vi "Robot Global Data.vi"() -> ()   [LabVIEW 2015]
doc: "This global VI can contain as many global variables as you need. Place a control on the panel, give it a good name. To read or write to it from a VI, drag the icon to the diagram of that VI. You can also drag from the project. Click on the node to change which global you access. You shouldn't have multiple locations writing to a global or it will cause a race-condition."
uses:
  <vilib>/Rock Robotics/WPI/Camera/WPI_CameraImageSize.ctl
  <vilib>/Rock Robotics/WPI/DriverStation/WPI_DriverStationRobotMode2.ctl
  02042014LargeBallRobot/010214-Dashboard-TMJB/Program Files (x86)/National Instruments/LabVIEW 2013/examples/FRC/Vision/2014 Target Detection/TargetType.ctl
panel:
  out "Arcade y":dbl
  out "Arcade x":dbl
  out "Tank Right":dbl
  out "Tank Left":dbl
  in  "MasterSolenoidOut":bool
  in  "MasterSolenoidIn":bool
  in  "FlappyWingsOut":bool
  in  "FlappyWingsIn":bool
  in  "AutoMove":T1(ring)
  in  "Current Speed":cluster{"Left":dbl, "Right":dbl}
  in  "DriveBaseControls":T2
  in  "ArmReverse":bool
  in  "ArmForward":bool
  in  "intakeSpeed":dbl
  in  "AutoTarget":T4
  in  "Robot Mode":T5
  in  "LED toggle rate (ms)":u32=20
  in  "image size":T6=enum."320x240"
  in  "Enable Vision":bool
  # "Payload Controls"
  # "Arcade Drive Indicators"
  # "Tank Drive Indicators"
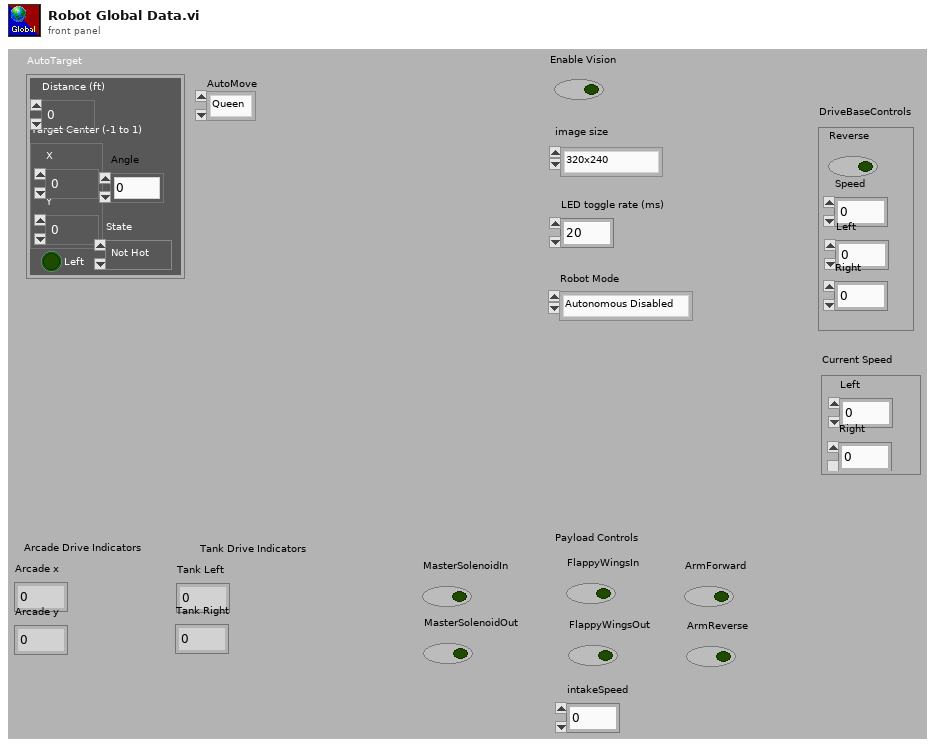
[diagram p1: front panel]
types:
  T1 = enum16{"Queen", "King", "Rook", "Knight", "Pawn"}
  T2 = cluster{"Reverse":bool, "Speed":dbl, "Left":dbl, "Right":dbl}
  T3 = typedef "TargetType.ctl" = enum16{"Not Hot", "Hot"}
  T4 = cluster{"Distance (ft)":dbl, "Target Center (-1 to 1)":cluster{"X":dbl, "Y":dbl}, "Left":bool, "State":T3, "Angle":dbl}
  T5 = typedef "WPI_DriverStationRobotMode2.ctl" = enum16{"Autonomous Disabled", "Autonomous Enabled", "Teleop Disabled", "Teleop Enabled", "Disconnected", "Finish", "Test Disabled", "Test Enabled"}
  T6 = typedef "WPI_CameraImageSize.ctl" = enum16{"640x480", "320x240", "160x120"}
diagram:
